vi "Example - Cluster Advanced retrieve rulers.vi"() -> ()   [LabVIEW 2017]
uses:
  da318448-3cad-42ed-b567-b1a7b9d2dcdc.vi
  8b979ef5-f5f6-4d36-b0d8-cf42d7dfdfe2.vi
  0333efe5-f0fb-4901-b6dd-db031cec30c6.vi
  API-String-Arugments-Support/_Support/Convert API String Arguments to Data(variant).vi
panel:
  out "[output cluster]":T1(array[cluster])=[{"String"="{BoolArray:[0,1,0,1;1,0,1,0;0,1,0,1];Cluster.Boolean:True}", "Reference Cluster"={"String"="abc", "BoolArray"=[[TRUE, FALSE, TRUE, FALSE], [FALSE, TRUE, FALSE, TRUE], [TRUE, FALSE, TRUE, FALSE]], "Cluster"={"Boolean"=FALSE}}, "Retrieved Cluster"={"String"="abc", "BoolArray"=[[FALSE, TRUE, FALSE, TRUE], [TRUE, FALSE, TRUE, FALSE], [FALSE, TRUE, FALSE, TRUE]], "Cluster"={"Boolean"=TRUE}}}, {"String"="BoolArray:[TRUE,FALSE,TRUE,FALSE;FALSE,TRUE,FALSE,TRUE;TRUE,FALSE,TRUE,FALSE];Cluster.Boolean:off", "Reference Cluster"={"String"="def", "BoolArray"=[[FALSE, TRUE, FALSE, TRUE], [TRUE, FALSE, TRUE, FALSE], [FALSE, TRUE, FALSE, TRUE]], "Cluster"={"Boolean"=TRUE}}, "Retrieved Cluster"={"String"="def", "BoolArray"=[[TRUE, FALSE, TRUE, FALSE], [FALSE, TRUE, FALSE, TRUE], [TRUE, FALSE, TRUE, FALSE]], "Cluster"={"Boolean"=FALSE}}}]
  out "output cluster":T2={"String"="{BoolArray:[TRUE,FALSE,TRUE,FALSE;FALSE,TRUE,FALSE,TRUE;TRUE,FALSE,TRUE,FALSE];Cluster.Boolean:True}", "Reference Cluster"={"String"="abc", "BoolArray"=[[FALSE, TRUE, FALSE, TRUE], [TRUE, FALSE, TRUE, FALSE], [FALSE, TRUE, FALSE, TRUE]], "Cluster"={"Boolean"=FALSE}}, "Retrieved Cluster"={"String"="abc", "BoolArray"=[[TRUE, FALSE, TRUE, FALSE], [FALSE, TRUE, FALSE, TRUE], [TRUE, FALSE, TRUE, FALSE]], "Cluster"={"Boolean"=TRUE}}}
  out "output cluster 2":T3={"String"="[{BoolArray:[0,1,0,1;1,0,1,0;0,1,0,1];Cluster.Boolean:True},{BoolArray:[TRUE,FALSE,TRUE,FALSE;FALSE,TRUE,FALSE,TRUE;TRUE,FALSE,TRUE,FALSE]}]", "Reference Cluster Array"=[{"String"="abc", "BoolArray"=[[TRUE, FALSE, TRUE, FALSE], [FALSE, TRUE, FALSE, TRUE], [TRUE, FALSE, TRUE, FALSE]], "Cluster"={"Boolean"=FALSE}}, {"String"="def", "BoolArray"=[[FALSE, TRUE, FALSE, TRUE], [TRUE, FALSE, TRUE, FALSE], [FALSE, TRUE, FALSE, TRUE]], "Cluster"={"Boolean"=TRUE}}], "Retrieved Cluster Array"=[{"String"="", "BoolArray"=[[FALSE, TRUE, FALSE, TRUE], [TRUE, FALSE, TRUE, FALSE], [FALSE, TRUE, FALSE, TRUE]], "Cluster"={"Boolean"=TRUE}}, {"String"="", "BoolArray"=[[TRUE, FALSE, TRUE, FALSE], [FALSE, TRUE, FALSE, TRUE], [TRUE, FALSE, TRUE, FALSE]], "Cluster"={"Boolean"=FALSE}}]}
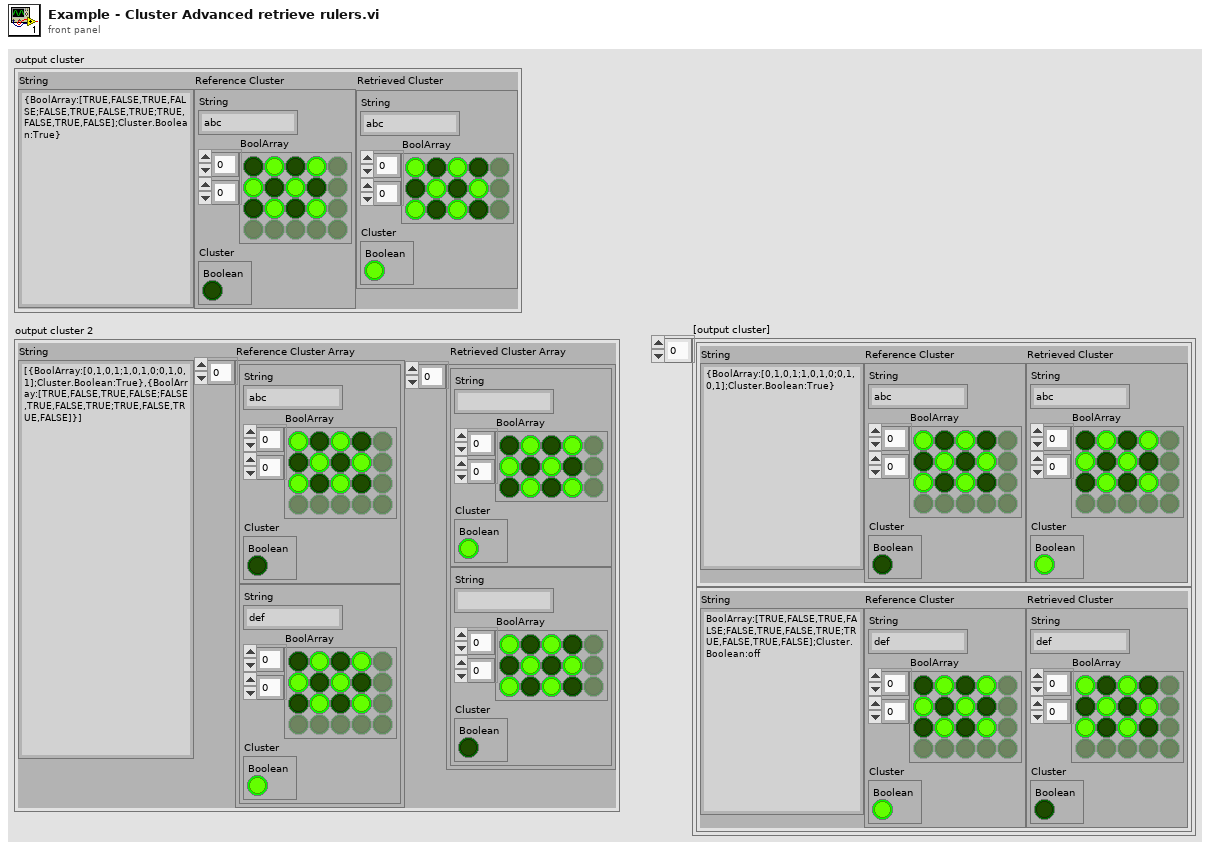
[diagram p1: front panel]
types:
  T1 = cluster{"String":string, "Reference Cluster":cluster{"String":string, "BoolArray":bool[][], "Cluster":cluster{"Boolean":bool}}, "Retrieved Cluster":cluster{"String":string, "BoolArray":bool[][], "Cluster":cluster{"Boolean":bool}}}[]
  T2 = cluster{"String":string, "Reference Cluster":cluster{"String":string, "BoolArray":bool[][], "Cluster":cluster{"Boolean":bool}}, "Retrieved Cluster":cluster{"String":string, "BoolArray":bool[][], "Cluster":cluster{"Boolean":bool}}}
  T3 = cluster{"String":string, "Reference Cluster Array":cluster{"String":string, "BoolArray":bool[][], "Cluster":cluster{"Boolean":bool}}[], "Retrieved Cluster Array":cluster{"String":string, "BoolArray":bool[][], "Cluster":cluster{"Boolean":bool}}[]}
  T4 = cluster{"String":string, "BoolArray":bool[][], "Cluster":cluster{"Boolean":bool}}
  T5 = cluster{"String":string, "BoolArray":bool[][], "Cluster":cluster{"Boolean":bool}}[]
  T6 = cluster{"String":string, "Cluster":cluster{"String":string, "BoolArray":bool[][], "Cluster":cluster{"Boolean":bool}}[], "Data":cluster{"String":string, "BoolArray":bool[][], "Cluster":cluster{"Boolean":bool}}[]}
  T7 = cluster{"String":string, "Cluster":cluster{"String":string, "BoolArray":bool[][], "Cluster":cluster{"Boolean":bool}}, "Data":cluster{"String":string, "BoolArray":bool[][], "Cluster":cluster{"Boolean":bool}}}
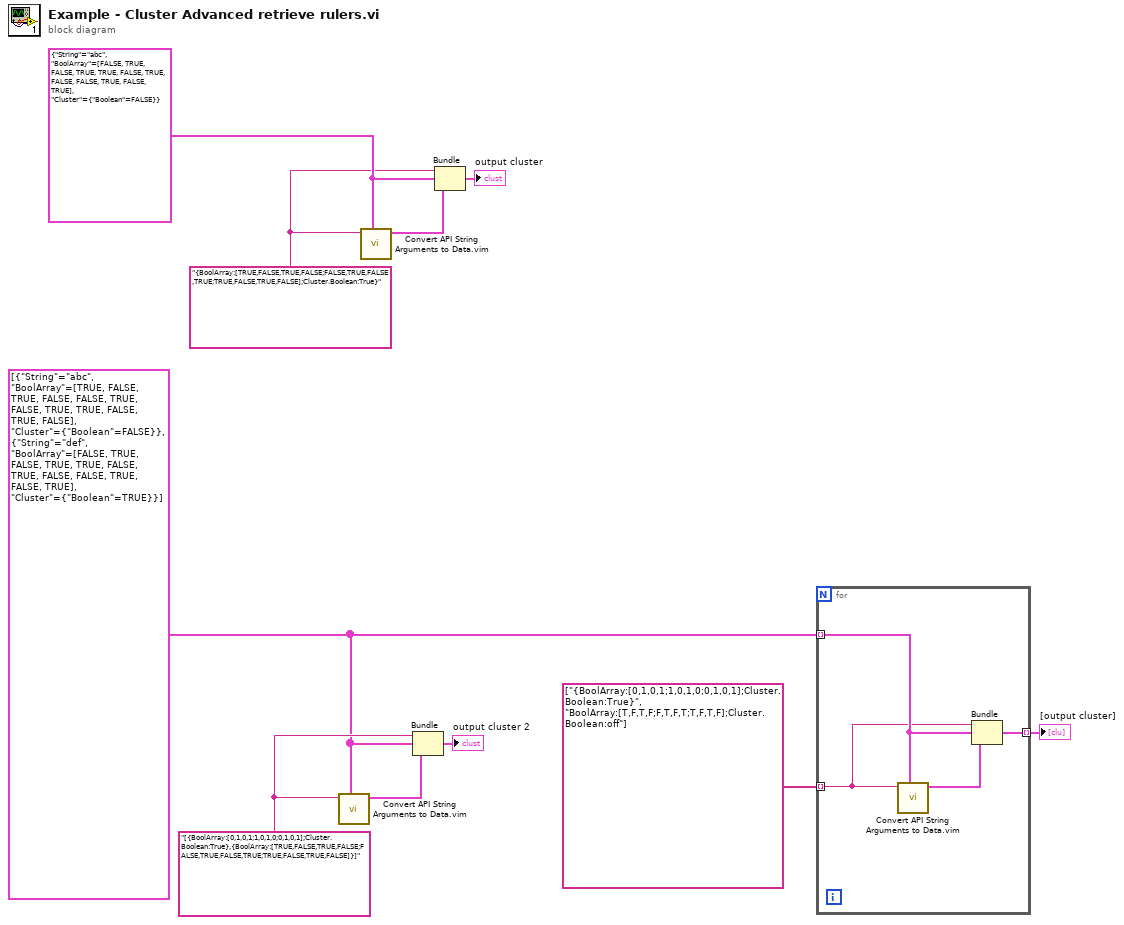
[diagram p0: block diagram]
diagram:
  w4 = "{BoolArray:[TRUE,FALSE,TRUE,FALSE;FALSE,TRUE,FALSE,TRUE;TRUE,FALSE,TRUE,FALSE];Cluster.Boolean:True}" ("String")
  w5 = T4 {"String"="abc", "BoolArray"=[[FALSE, TRUE, FALSE, TRUE], [TRUE, FALSE, TRUE, FALSE], [FALSE, TRUE, FALSE, TRUE]], "Cluster"={"Boolean"=FALSE}} ("Cluster")
  w10 = "[{BoolArray:[0,1,0,1;1,0,1,0;0,1,0,1];Cluster.Boolean:True},{BoolArray:[TRUE,FALSE,TRUE,FALSE;FALSE,TRUE,FALSE,TRUE;TRUE,FALSE,TRUE,FALSE]}]" ("String")
  w3 = T5 [{"String"="abc", "BoolArray"=[[TRUE, FALSE, TRUE, FALSE], [FALSE, TRUE, FALSE, TRUE], [TRUE, FALSE, TRUE, FALSE]], "Cluster"={"Boolean"=FALSE}}, {"String"="def", "BoolArray"=[[FALSE, TRUE, FALSE, TRUE], [TRUE, FALSE, TRUE, FALSE], [FALSE, TRUE, FALSE, TRUE]], "Cluster"={"Boolean"=TRUE}}] ("Cluster")
  n1 = call "Convert API String Arguments to Data.vim"("Type"=w3, "String"=w10) -> ("Data"=w9:T5)  [unwired: 6 in, 1 out]
  n2 = call "Convert API String Arguments to Data.vim"("Type"=w5, "String"=w4) -> ("Data"=w6:T4)  [unwired: 6 in, 1 out]
  n3 = Bundle("String"=w10, "Cluster"=w3, "Data"=w9) -> (→"output cluster 2":T6)  [unwired: 1 in]
  n4 = Bundle("String"=w4, "Cluster"=w5, "Data"=w6) -> (→"output cluster":T7)  [unwired: 1 in]
  n5 = for {
    tunnel: w3 -> [w13] mode=indexing
    tunnel: string[] ["{BoolArray:[0,1,0,1;1,0,1,0;0,1,0,1];Cluster.Boolean:True}", "BoolArray:[TRUE,FALSE,TRUE,FALSE;FALSE,TRUE,FALSE,TRUE;TRUE,FALSE,TRUE,FALSE];Cluster.Boolean:off"] ("String") -> [w12] mode=indexing
    tunnel: [w11] -> w1 mode=indexing
    n6 = call "Convert API String Arguments to Data.vim"("Type"=w13, "String"=w12) -> ("Data"=w14:T4)  [unwired: 6 in, 1 out]
    n7 = Bundle("String"=w12, "Cluster"=w13, "Data"=w14) -> (w11:T7)  [unwired: 1 in]
  }
  "[output cluster]" <- w1
